vi "Load Speed Data.vi"(8 "error in (no error)":errorcluster, 11 "AVI File Path":path) -> (0 "error out":errorcluster, 3 "Speed Data":string[][](array[string]))   [LabVIEW 2017]
uses:
  <userlib>/My Palettes.lib/Files & paths/Spreadsheet/Read From Spreadsheet File (string)-Mod.vi
panel:
  out "Speed data file found":bool
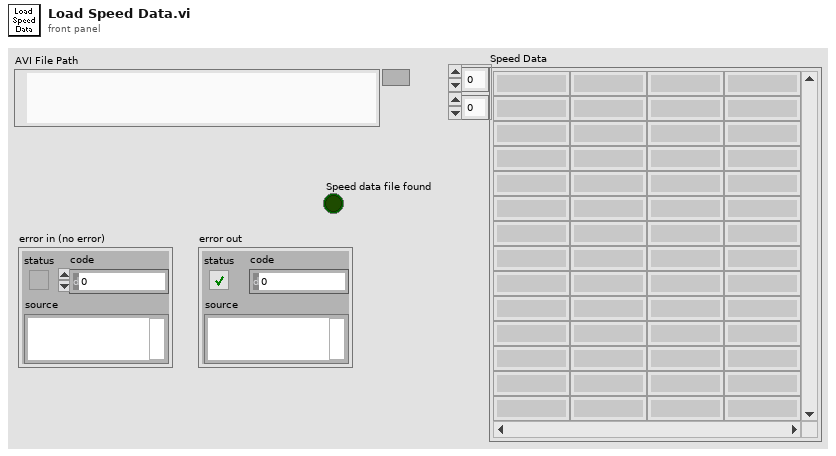
[diagram p1: front panel]
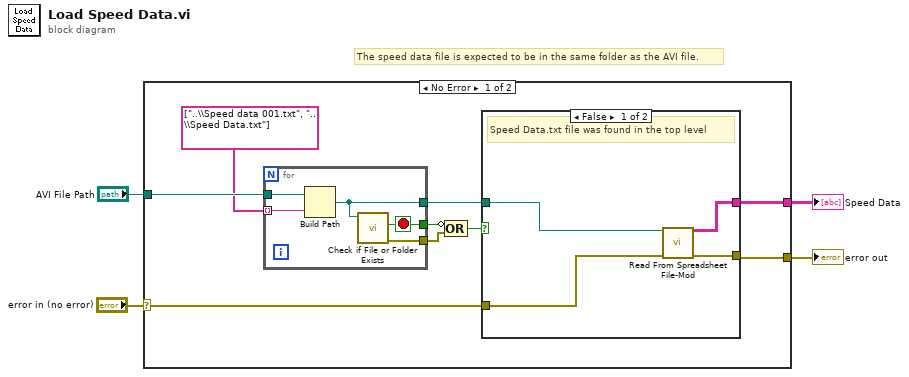
[diagram p0: block diagram]
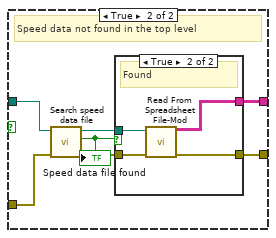
[diagram p2: hidden frame]
diagram:
  # "The speed data file is expected to be in the same folder as the AVI file."
  n1 = case shown="No Error" "error in (no error)" {
    selector: "error in (no error)" -> [w6 w35]
    tunnel: "AVI File Path" -> [w13 _]
    tunnel: [w12 _] -> w3
    tunnel: [w7 w35] -> w2
    frame No Error {
      n2 = for {
        tunnel: w13 -> [w18]
        tunnel: [w17] -> w11
        tunnel: [w16] -> w10
        tunnel: [w14] -> w9
        tunnel: string[] ["..\\Speed data 001.txt", "..\\Speed Data.txt"] -> [w15] mode=indexing
        stop <- w14 stop-if-true
        n3 = Build Path(base path=w18, name or relative path=w15) -> (appended path=w17:path)
        n4 = call <vilib>:"Check if File or Folder Exists.vi"("path"=w17) -> ("error out"=w16:errorcluster, "file or folder exists?"=w14:bool)  [unwired: 8 in, 1 out]
      }
      n5 = Compound Arithmetic op=OR(invert w9, w10) -> (w8:bool)
      n6 = case shown="False" w8 {
        tunnel: w11 -> [w22 w28]
        tunnel: [w21 w24] -> w12
        tunnel: [w20 w26] -> w7
        tunnel: w6 -> [w19 w29]
        frame False {
          # "Speed Data.txt file was found in the top level"
          n7 = call-poly <userlib>:"Read From Spreadsheet File-Mod.vi"("file path (dialog if empty)"=w22, "error in"=w19) -> ("all rows"=w21:string[][], "error out"=w20:errorcluster)  [unwired: 8 in, 4 out]
        }
        frame True {
          # "Speed data not found in the top level"
          n8 = call "Search speed data file.vi"("error in (no error)"=w29, "Dummy AVI folder path"=w28) -> ("error out"=w27:errorcluster, "Speed data file found"=w23:bool, "1st speed data file's path"=w25:path)  [unwired: 7 in]
          "Speed data file found" <- w23
          n9 = case shown="True" w23 {
            tunnel: w27 -> [w30 w34]
            tunnel: [w30 w33] -> w26
            tunnel: w25 -> [_ w32]
            tunnel: [_ w31] -> w24
            frame False {
              # "Not found"
            }
            frame True {
              # "Found"
              n10 = call-poly <userlib>:"Read From Spreadsheet File-Mod.vi"("file path (dialog if empty)"=w32, "error in"=w34) -> ("all rows"=w31:string[][], "error out"=w33:errorcluster)  [unwired: 8 in, 4 out]
            }
          }
        }
      }
    }
    frame Error {
    }
  }
  "Speed Data" <- w3
  "error out" <- w2
